vi "NT Server.vi"(6 "Update Time":i32=100, 7 "Logging Config":T1={"Enable"=FALSE, "Log Path"=path "", "Log Flush (s)"=0.25}, 8 "error in (no error)":errorcluster, 9 "preloads":string[](array[string])=[""], 10 "Server Name":string="Robot", 11 "Enable Read Errors":bool) -> (0 "error out":errorcluster)   [LabVIEW 2025]
doc: "This VI runs the Network Table services for the robot. The top level of Robot Main is a good location. You may then read and write variables and they will be shared with Network Table clients."
uses:
  <vilib>/Rock Robotics/Network Tables/NT Globals.vi
  FRC_NetworkTablesLV.dll
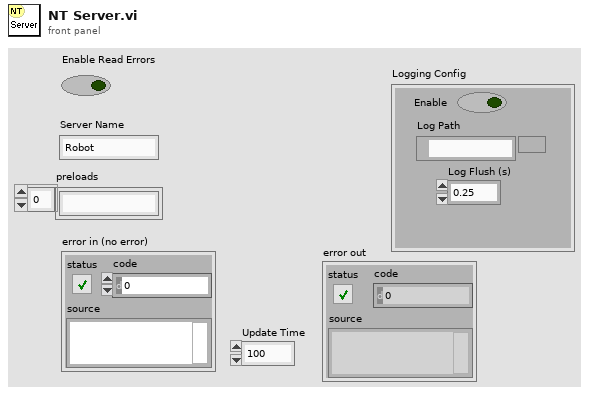
[diagram p1: front panel]
types:
  T1 = cluster{"Enable":bool, "Log Path":path, "Log Flush (s)":dbl}
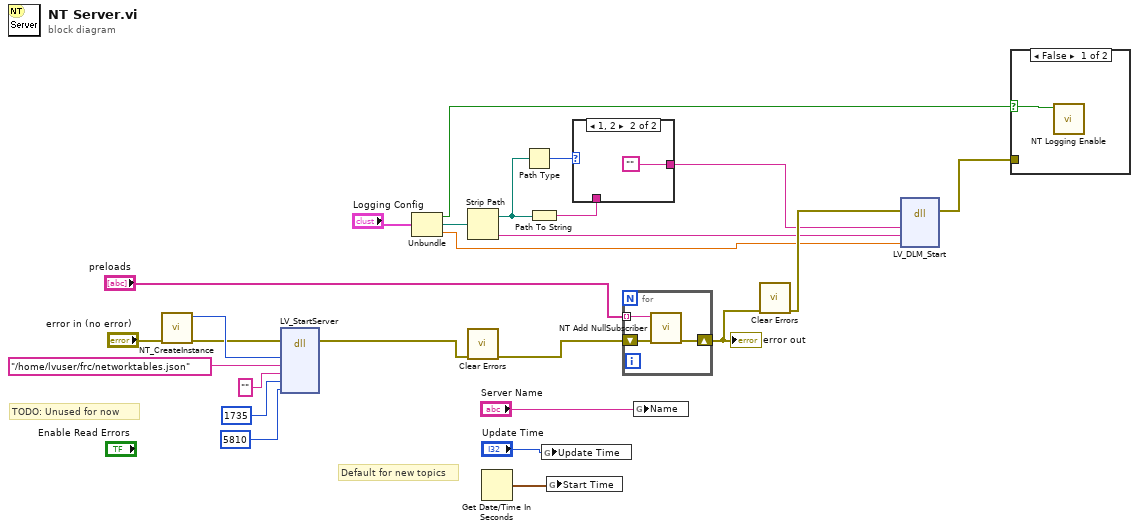
[diagram p0: block diagram]
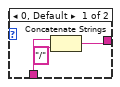
[diagram p3: hidden frame]
diagram:
  # "TODO: Unused for now"
  # "Default for new topics"
  n1 = call <vilib>:"NT_CreateInstance.vi"("error in (no error)"="error in (no error)") -> ("error out"=w20:errorcluster, "InstanceHandle"=w25:u64)  [unwired: 9 in]
  n2 = dll-call lib="FRC_NetworkTablesLV.*" fn="LV_StartServer"(error in=w20, "InstHandle"=w25, "persistFileName"="/home/lvuser/frc/networktables.json", "listenAddr"="", "port3"=u16 1735 ("port"), "port4"=u16 5810 ("port")) -> (error out=w13:errorcluster)  [unwired: 8 in, 1 out]
  n3 = Unbundle("Logging Config") -> ("Enable"=w6:bool, "Log Path"=w9:path, "Log Flush (s)"=w8:dbl)
  n4 = Strip Path(path=w9) -> (stripped path=w5:path, name=w7:string)
  n5 = call <vilib>:"Clear Errors.vi"("error in (no error)"=w13) -> ("error out"=w15:errorcluster)  [unwired: 5 in, 1 out]
  n6 = Get Date/Time In Seconds() -> (seconds since 1Jan1904=w17:timestamp)
  n7 = Path Type(1:w5) -> (0:w4:i16)
  n8 = Path To String(path=w5) -> (string=w3:string)
  n9 = global write "NT Globals.vi" "Update Time"("Update Time") -> ()
  n10 = global write "NT Globals.vi" "Start Time"(w17) -> ()
  n11 = case shown="1, 2" w4 {
    tunnel: [w26 ""] -> w2
    tunnel: w3 -> [w28 _]
    frame 0, Default {
      n12 = Concatenate Strings(w28, "/" ("string")) -> (w26:string)
    }
    frame 1, 2 {
    }
  }
  n13 = for {
    shift-right: [w31] -> w12
    shift-left: w15 -> [w32]
    tunnel: "preloads" -> [w30] mode=indexing
    n14 = call <vilib>:"NT Add NullSubscriber.vi"("error in (no error)"=w32, "match Pattern"=w30) -> ("error out"=w31:errorcluster)  [unwired: 9 in]
  }
  "error out" <- w12
  n15 = global write "NT Globals.vi" "Name"("Server Name") -> ()
  n16 = call <vilib>:"Clear Errors.vi"("error in (no error)"=w12) -> ("error out"=w11:errorcluster)  [unwired: 5 in, 1 out]
  n17 = dll-call lib="FRC_NetworkTablesLV.*" fn="LV_DLM_Start"(error in=w11, "dir"=w2, "name"=w7, "period(s)"=w8) -> (error out=w1:errorcluster)  [unwired: 6 in, 1 out]
  n18 = case shown="False" w6 {
    selector: w6 -> [w33 _]
    tunnel: w1 -> [_ _]
    frame False {
      n19 = call <vilib>:"NT Logging Enable.vi"("Enable"=w33) -> ()  [unwired: 11 in]
    }
    frame True {
      # "default is on"
    }
  }
